vi "Calib_Analyse_fit.vi"(0 "Calib file":path, 1 "Input points":dbl[][](array[numeric]) format="%.2f", 2 "polynomial order":i32=2, 5 "Fixed n":bool=TRUE, 7 "n":dbl=0.45 format="%.2f", 9 "Point selector 3":cluster{"Y":dbl, "X":dbl, "t/f":bool}[](array[cluster]) {"X" format="%.2f"; "Y" format="%.2f"}, 11 "Point selector 4":T1(array[cluster])=[{"Y"=3.5155385742, "Y2"=3.2773117676, "X"=-15.0, "t/f"=FALSE}, {"Y"=3.4946367187, "Y2"=3.3075422363, "X"=-10.0, "t/f"=FALSE}, {"Y"=3.473232666, "Y2"=3.3353713379, "X"=-5.0, "t/f"=FALSE}, {"Y"=3.454592041, "Y2"=3.3658986816, "X"=0.0, "t/f"=FALSE}, {"Y"=3.4246572266, "Y2"=3.3874455566, "X"=5.0, "t/f"=FALSE}, {"Y"=3.398965332, "Y2"=3.4137351074, "X"=10.0, "t/f"=FALSE}, {"Y"=3.362712646484375, "Y2"=3.428485595703125, "X"=15.0, "t/f"=FALSE}] {"Y2" format="%.2f"; "X" format="%.2f"; "Y" format="%.2f"}) -> (4 "Calib const":string[][](array[string])=[["n", "0.405000"], ["A", "7.730378"], ["B", "6.204067"], ["Av % err", "0.204301"]], 6 "Calibration plot":cluster{cluster{dbl, dbl}[]}[](graph)=[{[{0.8450215822560672, 12.972948762710196}, {0.9063644870167936, 13.35352428024258}, {1.0129933166229186, 14.015056729178777}, {1.0924501688964157, 14.50801239851709}, {1.2215481063301497, 15.308944707524116}, {1.3521910897315237, 16.119462585897956}, {1.4772434835777744, 16.895296069694275}]}, {[{0.8450215822560672, 12.97084622363197}, {0.9063644870167936, 13.353228276297402}, {1.0129933166229186, 14.026771757587431}, {1.0924501688964157, 14.499243467101884}, {1.2215481063301497, 15.307992219000921}, {1.3521910897315237, 16.116882250583185}, {1.4772434835777744, 16.898281339562185}]}], 8 "Average Temp":dbl=19.0 format="%.2f", 10 "Point selector 3 out":cluster{"Y":dbl, "X":dbl, "t/f":bool}[](array[cluster]) {"X" format="%.2f"; "Y" format="%.2f"}, 14 "Coefficients":dbl[][](array[numeric]) format="%.2f", 15 "Point selector 4 out":T1(array[cluster])=[{"Y"=3.5155385742, "Y2"=3.2773117676, "X"=-15.0, "t/f"=FALSE}, {"Y"=3.4946367187, "Y2"=3.3075422363, "X"=-10.0, "t/f"=FALSE}, {"Y"=3.473232666, "Y2"=3.3353713379, "X"=-5.0, "t/f"=FALSE}, {"Y"=3.454592041, "Y2"=3.3658986816, "X"=0.0, "t/f"=FALSE}, {"Y"=3.4246572266, "Y2"=3.3874455566, "X"=5.0, "t/f"=FALSE}, {"Y"=3.398965332, "Y2"=3.4137351074, "X"=10.0, "t/f"=FALSE}, {"Y"=3.362712646484375, "Y2"=3.428485595703125, "X"=15.0, "t/f"=FALSE}] {"Y2" format="%.2f"; "X" format="%.2f"; "Y" format="%.2f"})   [LabVIEW 2010]
uses:
  Globals/Calib_global.vi
  Acquisition/PWA/PWAtasksGLOBAL.vi
  <vilib>/Analysis/NI_AALBase.lvlib
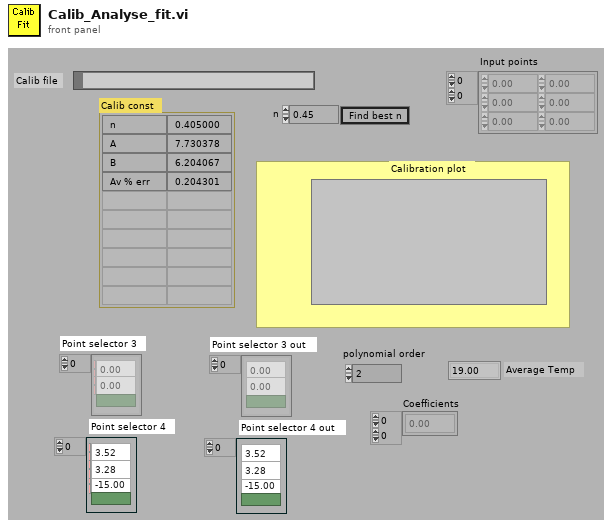
[diagram p1: front panel]
types:
  T1 = cluster{"Y":dbl, "Y2":dbl, "X":dbl, "t/f":bool}[]
  T2 = typedef "Cal_Inst_type.ctl" = enum16{"Propeller anemometer", "Pressure Transducer", "Hot wire", "Cross wire velocity", "Cross wire angle", "Generic Linear", "Generic Polynomial", "Generic BackPoly", "Fast FID", "Thermocouple", "Cold wire", "Pulsed Wire"}
  T3 = cluster{"Y":dbl, "Y":dbl, "X":dbl, "switch":bool}
  T4 = typedef "Ref_Inst_type.ctl" = enum16{"Propellor anemometer", "Pressure Transducer", "Raw voltage", "Pitot-static tube", "Preston tube", "Generic Linear", "Generic Polynomial", "Thermocouple", "LDA", "Enter Value", "ADAM Channel"}
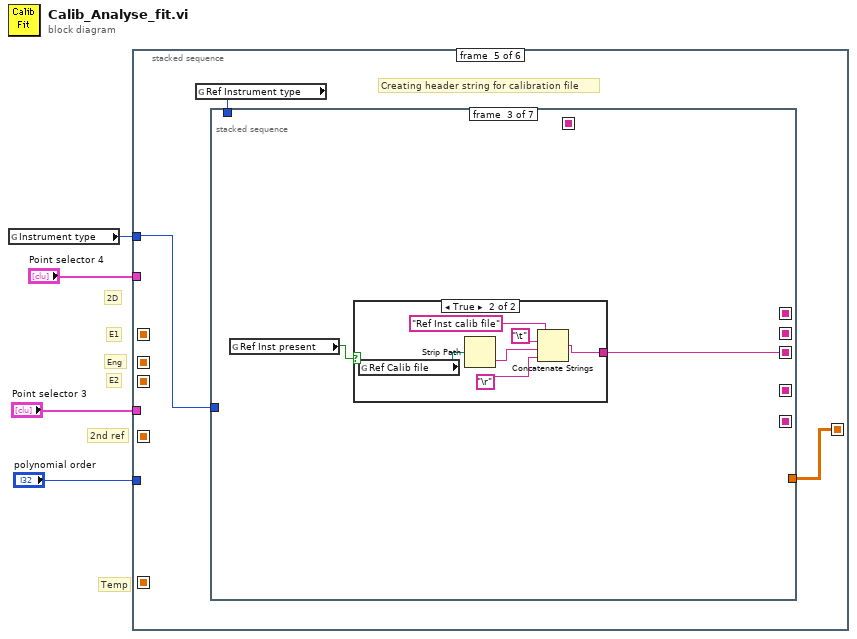
[diagram p0: block diagram]
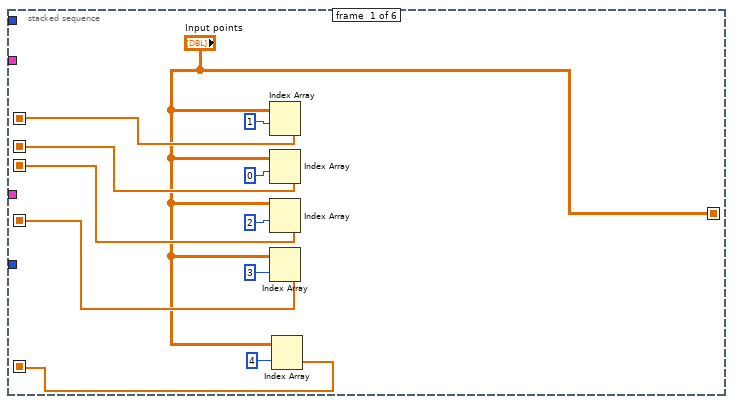
[diagram p2: hidden frame]
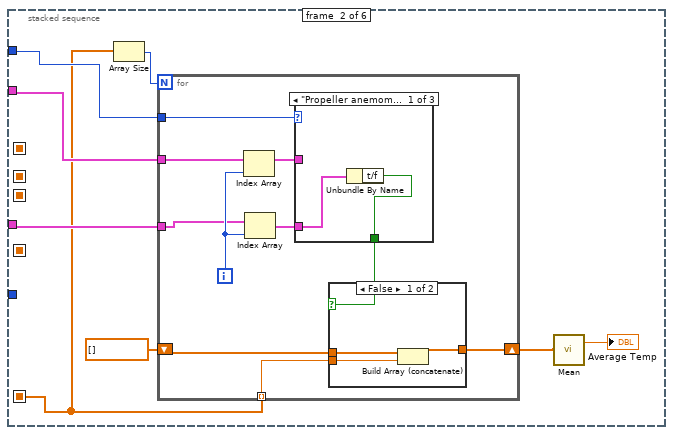
[diagram p3: hidden frame]
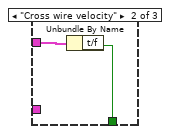
[diagram p5: hidden frame]
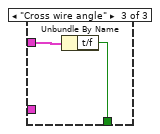
[diagram p6: hidden frame]
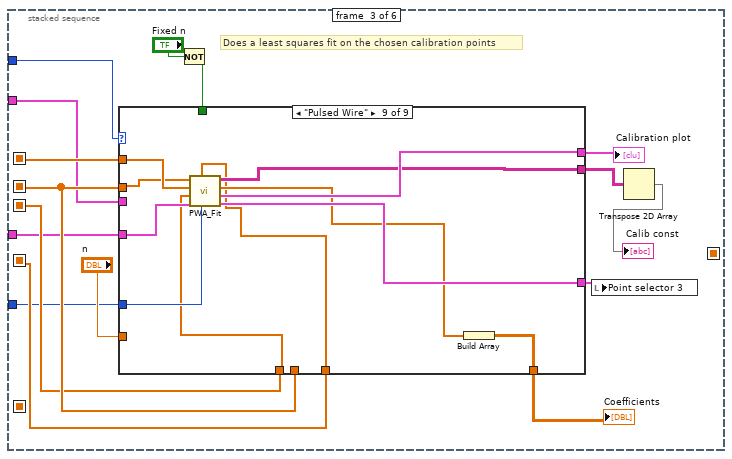
[diagram p7: hidden frame]
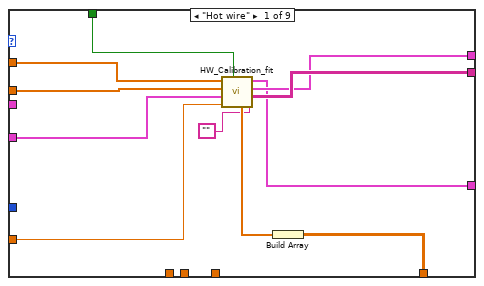
[diagram p8: hidden frame]
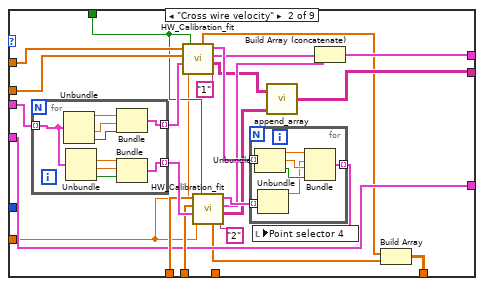
[diagram p9: hidden frame]
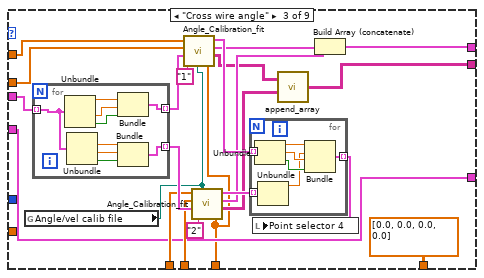
[diagram p10: hidden frame]
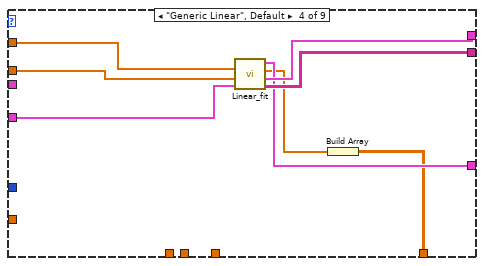
[diagram p11: hidden frame]
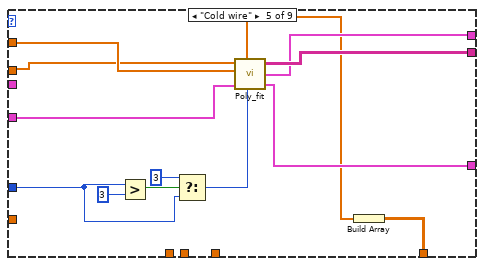
[diagram p12: hidden frame]
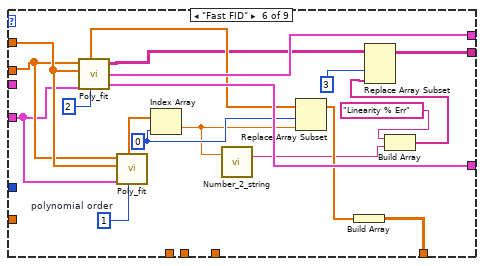
[diagram p13: hidden frame]
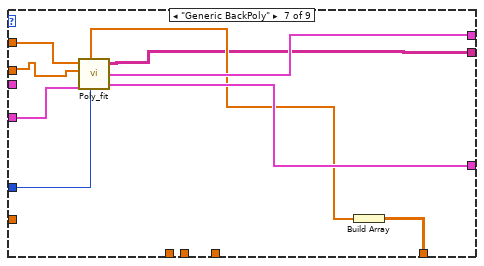
[diagram p14: hidden frame]
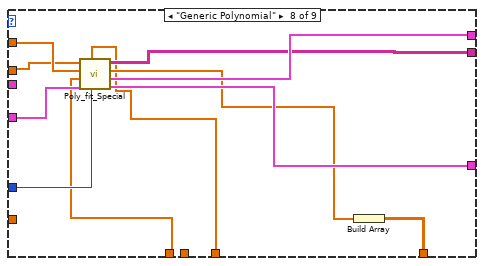
[diagram p15: hidden frame]
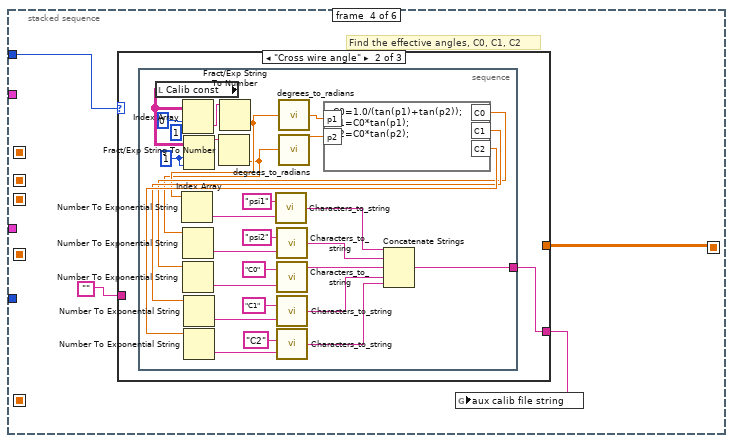
[diagram p16: hidden frame]
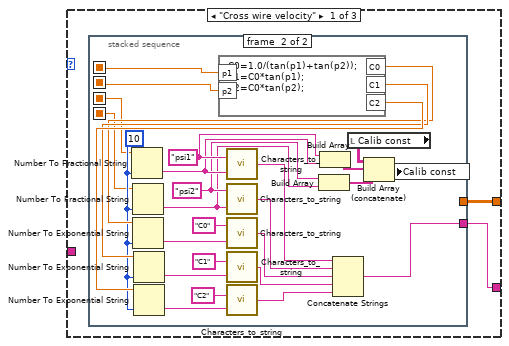
[diagram p17: hidden frame]
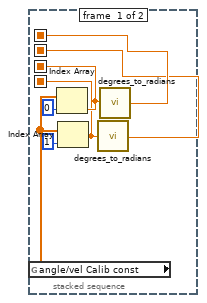
[diagram p18: hidden frame]
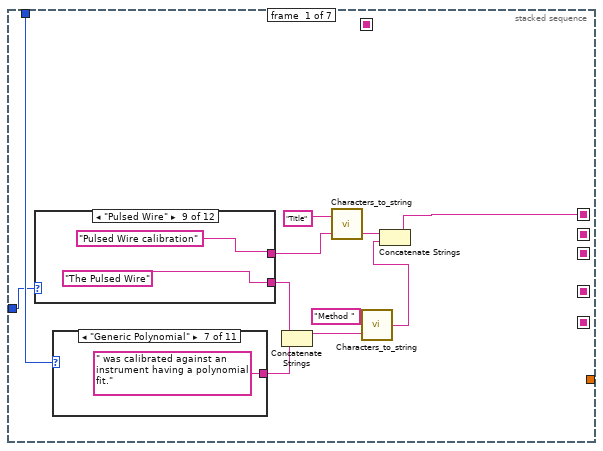
[diagram p20: hidden frame]
diagram:
  # "Temp"
  # "2D"
  # "2nd ref"
  # "E2"
  # "E1"
  # "Eng"
  n1 = global read "Calib_global.vi" "Instrument type"() -> (w4:T2)
  n2 = stacked-sequence {
    seq-local: ["Input points" _ _ _ _ _] -> [_ _ _ w221 w293 _]
    seq-local: [w11 _ _ _ _ _] -> [_ _ w52 _ _ _]
    seq-local: [w10 _ _ _ _ _] -> [_ _ w51 _ _ _]
    seq-local: [w9 _ _ _ _ _] -> [_ _ w50 _ _ _]
    seq-local: [w8 _ _ _ _ _] -> [_ _ w49 _ _ _]
    seq-local: [w5 _ _ _ _ _] -> [_ w17 _ _ _ _]
    tunnel: w4 -> [_ w23 w46 w220 w292 _]
    tunnel: "Point selector 3" -> [_ w22 w48 _ _ _]
    tunnel: "Point selector 4" -> [_ w21 w47 _ _ _]
    tunnel: "polynomial order" -> [_ _ w44 _ _ _]
    frame #0 {
      n3 = Index Array(array="Input points", index (row)=1) -> (element=w11:dbl[])  [unwired: 1 in]
      n4 = Index Array(array="Input points", index (row)=0) -> (element=w10:dbl[])  [unwired: 1 in]
      n5 = Index Array(array="Input points", index (row)=2) -> (element=w9:dbl[])  [unwired: 1 in]
      n6 = Index Array(array="Input points", index (row)=3) -> (element=w8:dbl[])  [unwired: 1 in]
      n7 = Index Array(array="Input points", index (row)=4) -> (element=w5:dbl[])  [unwired: 1 in]
    }
    frame #1 {
      n8 = Array Size(array=w17) -> (size(s)=w16:i32)
      n9 = for {
        N: w16 -> [_]
        tunnel: w23 -> [w33]
        tunnel: w22 -> [w25]
        tunnel: w21 -> [w27]
        shift-right: [w30] -> w18
        shift-left: dbl[] [] -> [w31]
        tunnel: w17 -> [w29] mode=indexing
        i -> [w26]
        n10 = Index Array(array=w27, index=w26) -> (element=w28:cluster{"Y":dbl, "Y2":dbl, "X":dbl, "t/f":bool})
        n11 = Index Array(array=w25, index=w26) -> (element=w24:cluster{"Y":dbl, "X":dbl, "t/f":bool})
        n12 = case shown="\"Propeller anemometer\", Default" w33 {
          tunnel: w24 -> [w39 _ _]
          tunnel: w28 -> [_ w41 w43]
          tunnel: [w38 w40 w42] -> w32
          frame "Propeller anemometer", Default {
            n13 = Unbundle By Name(w39) -> ("t/f"=w38:bool)
          }
          frame "Cross wire velocity" {
            n14 = Unbundle By Name(w41) -> ("t/f"=w40:bool)
          }
          frame "Cross wire angle" {
            n15 = Unbundle By Name(w43) -> ("t/f"=w42:bool)
          }
        }
        n16 = case shown="False" w32 {
          tunnel: w31 -> [w36 w37]
          tunnel: [w35 w37] -> w30
          tunnel: w29 -> [w34 _]
          frame False {
            n17 = Build Array (concatenate)(w36, w34) -> (w35:dbl[])
          }
          frame True {
          }
        }
      }
      n18 = call <vilib>:"Mean.vi"("X"=w18) -> ("mean"=→"Average Temp":dbl)  [unwired: 1 out]
    }
    frame #2 {
      # "Does a least squares fit on the chosen calibration points"
      n19 = Not(x="Fixed n") -> (.not. x?=w54:bool)
      n20 = case shown="\"Pulsed Wire\"" w46 {
        tunnel: [w65 w82 w120 w151 w166 w187 w196 w207 w218] -> w57
        tunnel: w52 -> [w70 w94 w132 w156 w165 w176 w193 w205 w216]
        tunnel: w51 -> [w69 w93 w131 w155 w164 w175 w192 w204 w215]
        tunnel: w54 -> [w68 w80 _ _ _ _ _ _ _]
        tunnel: w47 -> [_ w83 w121 _ _ _ _ _ _]
        tunnel: [w67 w76 w114 w154 w169 w177 w190 w201 w212] -> w55
        tunnel: [w66 w84 w122 w153 w168 w188 w197 w208 w219] -> w56
        tunnel: w51 -> [_ w89 w127 _ _ _ _ _ _]
        tunnel: w50 -> [_ w88 w126 _ _ _ _ w199 w210]
        tunnel: w48 -> [w64 w82 w120 w152 w167 w174 w194 w203 w214]
        tunnel: "n" -> [w63 w79 _ _ _ _ _ _ _]
        tunnel: w49 -> [_ _ w113 _ _ _ _ w198 w209]
        tunnel: [w61 w73 dbl[][] [[0.0, 0.0], [0.0, 0.0]] w149 w158 w186 w195 w206 w217] -> w45
        tunnel: w44 -> [_ _ _ _ w157 _ w189 w200 w211]
        frame "Hot wire" {
          n21 = call "HW_Calibration_fit.vi"("coeff suffix"="", "Fixed n (F)"=w68, "n input  (0.45)"=w63, "Point selector"=w64, "Velocity"=w69, "HW voltage"=w70) -> ("Calib const"=w67:string[][], "Calibration plot"=w66:cluster{cluster{dbl, "mse":dbl}[]}[], "Point selector"=w65:cluster{"Y":dbl, "X":dbl, "switch":bool}[], "Coefficients"=w62:dbl[])
          n22 = Build Array(w62) -> (w61:dbl[][])
        }
        frame "Cross wire velocity" {
          n23 = for {
            tunnel: w83 -> [w106] mode=indexing
            tunnel: [w107] -> w92 mode=indexing
            tunnel: [w105] -> w90 mode=indexing
            n24 = Unbundle(w106) -> ("Y"=w110:dbl, "X"=w109:dbl, "t/f"=w108:bool)  [unwired: 1 out]
            n25 = Unbundle(w106) -> ("Y2"=w104:dbl, "X"=w103:dbl, "t/f"=w102:bool)  [unwired: 1 out]
            n26 = Bundle("Y"=w110, "X"=w109, "t/f"=w108) -> (w107:cluster{"Y":dbl, "X":dbl, "t/f":bool})  [unwired: 1 out]
            n27 = Bundle("Y2"=w104, "X"=w103, "t/f"=w102) -> (w105:cluster{"Y2":dbl, "X":dbl, "t/f":bool})  [unwired: 1 out]
          }
          n28 = call "HW_Calibration_fit.vi"("coeff suffix"="1", "Fixed n (F)"=w80, "n input  (0.45)"=w79, "Point selector"=w92, "Velocity"=w93, "HW voltage"=w94) -> ("Calib const"=w77:string[][], "Calibration plot"=w85:cluster{cluster{dbl, "mse":dbl}[]}[], "Point selector"=w91:cluster{"Y":dbl, "X":dbl, "switch":bool}[], "Coefficients"=w71:dbl[])
          n29 = call "HW_Calibration_fit.vi"("coeff suffix"="2", "Fixed n (F)"=w80, "n input  (0.45)"=w79, "Point selector"=w90, "Velocity"=w89, "HW voltage"=w88) -> ("Calib const"=w78:string[][], "Calibration plot"=w86:cluster{cluster{dbl, "mse":dbl}[]}[], "Point selector"=w87:cluster{"Y":dbl, "X":dbl, "switch":bool}[], "Coefficients"=w72:dbl[])
          n30 = for {
            tunnel: w91 -> [w101] mode=indexing
            tunnel: [w97] -> w81 mode=indexing
            tunnel: w87 -> [w96] mode=indexing
            n31 = Unbundle(w101) -> ("Y"=w100:dbl, "X"=w99:dbl, "switch"=w98:bool)
            n32 = Unbundle(w96) -> ("Y"=w95:dbl)  [unwired: 2 out]
            n33 = Bundle("Y"=w100, "Y"=w95, "X"=w99, "switch"=w98) -> (w97:T3)  [unwired: 1 out]
          }
          n34 = local write "Point selector 4"(w81) -> ()
          n35 = call "append_array.vi"("array 2"=w78, "array 1"=w77) -> ("appended array"=w76:string[][])
          n36 = Build Array (concatenate)(w85, w86) -> (w84:cluster{cluster{dbl, "mse":dbl}[]}[])
          n37 = Build Array(w71, w72) -> (w73:dbl[][])
        }
        frame "Cross wire angle" {
          n38 = global read "Calib_global.vi" "Angle/vel calib file"() -> (w112:path)
          n39 = for {
            tunnel: w121 -> [w144] mode=indexing
            tunnel: [w145] -> w130 mode=indexing
            tunnel: [w143] -> w128 mode=indexing
            n40 = Unbundle(w144) -> ("Y"=w148:dbl, "X"=w147:dbl, "t/f"=w146:bool)  [unwired: 1 out]
            n41 = Unbundle(w144) -> ("Y2"=w142:dbl, "X"=w141:dbl, "t/f"=w140:bool)  [unwired: 1 out]
            n42 = Bundle("Y"=w148, "X"=w147, "t/f"=w146) -> (w145:cluster{"Y":dbl, "X":dbl, "t/f":bool})  [unwired: 1 out]
            n43 = Bundle("Y2"=w142, "X"=w141, "t/f"=w140) -> (w143:cluster{"Y2":dbl, "X":dbl, "t/f":bool})  [unwired: 1 out]
          }
          n44 = call "Angle_Calibration_fit.vi"("Reference Velocity"=w113, "Vel calib file"=w112, "coeff suffix"="1", "Point selector"=w130, "Angle"=w131, "HW voltage"=w132) -> ("Calib const"=w116:string[][], "Angle calibration (output)"=w123:cluster{cluster{"Y":dbl, "Y":dbl}[]}[], "Point selector"=w129:cluster{"Y":dbl, "X":dbl, "switch":bool}[])
          n45 = call "Angle_Calibration_fit.vi"("Reference Velocity"=w113, "Vel calib file"=w112, "coeff suffix"="2", "Point selector"=w128, "Angle"=w127, "HW voltage"=w126) -> ("Calib const"=w115:string[][], "Angle calibration (output)"=w124:cluster{cluster{"Y":dbl, "Y":dbl}[]}[], "Point selector"=w125:cluster{"Y":dbl, "X":dbl, "switch":bool}[])
          n46 = for {
            tunnel: w129 -> [w139] mode=indexing
            tunnel: [w135] -> w119 mode=indexing
            tunnel: w125 -> [w134] mode=indexing
            n47 = Unbundle(w139) -> ("Y"=w138:dbl, "X"=w137:dbl, "switch"=w136:bool)
            n48 = Unbundle(w134) -> ("Y"=w133:dbl)  [unwired: 2 out]
            n49 = Bundle("Y"=w138, "Y"=w133, "X"=w137, "switch"=w136) -> (w135:T3)  [unwired: 1 out]
          }
          n50 = local write "Point selector 4"(w119) -> ()
          n51 = call "append_array.vi"("array 2"=w115, "array 1"=w116) -> ("appended array"=w114:string[][])
          n52 = Build Array (concatenate)(w123, w124) -> (w122:cluster{cluster{"Y":dbl, "Y":dbl}[]}[])
        }
        frame "Generic Linear", Default {
          n53 = call "Linear_fit.vi"("Point selector"=w152, "Input X array"=w155, "Input Y array"=w156) -> ("Calib const"=w154:string[][], "Calibration plot"=w153:cluster{cluster{dbl, dbl}[]}[], "Coefficients"=w150:dbl[], "Point selector"=w151:cluster{"Y":dbl, "X":dbl, "switch":bool}[])  [unwired: 1 out]
          n54 = Build Array(w150) -> (w149:dbl[][])
        }
        frame "Cold wire" {
          n55 = Greater?(x=w157, y=3) -> (0:w162:bool)
          n56 = Select(t=3, s=w162, f=w157) -> (s? t:f=w160:i32)
          n57 = call "Poly_fit.vi"("Input Y array"=w164, "Input X array"=w165, "polynomial order"=w160, "Point selector"=w167) -> ("Coefficients"=w159:dbl[], "Calib const"=w169:string[][], "Calibration plot"=w168:cluster{cluster{dbl, dbl}[]}[], "Point selector"=w166:cluster{"Y":dbl, "X":dbl, "switch":bool}[])  [unwired: 1 out]
          n58 = Build Array(w159) -> (w158:dbl[][])
        }
        frame "Fast FID" {
          w181 = 0 ("index")
          w184 = 1  # polynomial order
          n59 = call "Poly_fit.vi"("Input Y array"=w175, "Input X array"=w176, "polynomial order"=2, "Point selector"=w174) -> ("Coefficients"=w182:dbl[], "Calib const"=w179:string[][], "Calibration plot"=w188:cluster{cluster{dbl, dbl}[]}[], "Point selector"=w187:cluster{"Y":dbl, "X":dbl, "switch":bool}[])  [unwired: 1 out]
          n60 = call "Poly_fit.vi"("Input Y array"=w175, "Input X array"=w176, "polynomial order"=w184, "Point selector"=w174) -> ("Coefficients"=w183:dbl[])  [unwired: 4 out]
          n61 = Index Array(array=w183, index=w181) -> (element=w173:dbl)
          n62 = call "Number_2_string.vi"("number"=w173) -> ("String"=w171:string)  [unwired: 1 in]
          n63 = Replace Array Subset(array=w182, new element=w173, index=w181) -> (w180:dbl[])
          n64 = Build Array(w180) -> (w186:dbl[][])
          n65 = Build Array("Linearity % Err" ("new element/subarray"), w171) -> (w170:string[])
          n66 = Replace Array Subset(array=w179, new element=w170, index (col)=3 ("disabled index (col)")) -> (w177:string[][])  [unwired: 1 in]
        }
        frame "Generic BackPoly" {
          n67 = call "Poly_fit.vi"("Input Y array"=w193, "Input X array"=w192, "polynomial order"=w189, "Point selector"=w194) -> ("Coefficients"=w191:dbl[], "Calib const"=w190:string[][], "Calibration plot"=w197:cluster{cluster{dbl, dbl}[]}[], "Point selector"=w196:cluster{"Y":dbl, "X":dbl, "switch":bool}[])  [unwired: 1 out]
          n68 = Build Array(w191) -> (w195:dbl[][])
        }
        frame "Generic Polynomial" {
          n69 = call "Poly_fit_Special.vi"("polynomial order"=w200, "Input X^3"=w198, "Point selector"=w203, "Input X^2"=w199, "Input X array"=w205, "Input Y array"=w204) -> ("Point selector"=w207:cluster{"Y":dbl, "X":dbl, "switch":bool}[], "Calibration plot"=w208:cluster{cluster{dbl, dbl}[]}[], "Coefficients"=w202:dbl[], "Calib const"=w201:string[][])
          n70 = Build Array(w202) -> (w206:dbl[][])
        }
        frame "Pulsed Wire" {
          n71 = call "PWA_Fit.vi"("polynomial order"=w211, "Input X^3"=w209, "Point selector"=w214, "Input X^2"=w210, "Input X array"=w216, "Input Y array"=w215) -> ("Point selector"=w218:cluster{"Y":dbl, "X":dbl, "switch":bool}[], "Calibration plot"=w219:cluster{cluster{dbl, dbl}[]}[], "Coefficients"=w213:dbl[], "Calib const"=w212:string[][])
          n72 = Build Array(w213) -> (w217:dbl[][])
        }
      }
      "Calibration plot" <- w56
      "Coefficients" <- w45
      n73 = local write "Point selector 3"(w57) -> ()
      n74 = Transpose 2D Array(2D array=w55) -> (transposed array=→"Calib const":string[][])
    }
    frame #3 {
      # "Find the effective angles, C0, C1, C2"
      n75 = case shown="\"Cross wire angle\"" w220 {
        tunnel: "" -> [_ _ w291]
        tunnel: [w225 w261 w291] -> w223
        tunnel: w221 -> [w224 _ _]
        frame "Cross wire velocity" {
          n76 = stacked-sequence {
            seq-local: [w230 _] -> [_ w236]
            seq-local: [w229 _] -> [_ w234]
            seq-local: [w228 _] -> [_ w235]
            seq-local: [w227 _] -> [_ w233]
            tunnel: [_ w246] -> w225
            tunnel: w224 -> [_ _]
            frame #0 {
              n77 = global read "Calib_global.vi" "angle/vel Calib const"() -> (w226:dbl[])
              n78 = Index Array(array=w226, index=0) -> (element=w228:dbl)
              n79 = Index Array(array=w226, index=1) -> (element=w227:dbl)
              n80 = call "degrees_to_radians.vi"("degrees"=w227) -> ("radians"=w229:dbl)
              n81 = call "degrees_to_radians.vi"("degrees"=w228) -> ("radians"=w230:dbl)
            }
            frame #1 {
              w237 = 10
              w243 = "psi2"
              w245 = "psi1"
              n82 = Number To Fractional String(number=w235, precision (6)=w237) -> (F-format string=w244:string)  [unwired: 2 out]
              n83 = Number To Fractional String(number=w233, precision (6)=w237) -> (F-format string=w242:string)  [unwired: 2 out]
              n84 = formula code="C0=1.0/(tan(p1)+tan(p2));\nC1=C0*tan(p1);\nC2=C0*tan(p2);"("p1"=w236, "p2"=w234) -> ("C0"=w258:dbl, "C1"=w259:dbl, "C2"=w260:dbl)
              n85 = Number To Exponential String(number=w258, precision (6)=w237) -> (E-format string=w256:string)  [unwired: 2 out]
              n86 = Number To Exponential String(number=w259, precision (6)=w237) -> (E-format string=w254:string)  [unwired: 2 out]
              n87 = Number To Exponential String(number=w260, precision (6)=w237) -> (E-format string=w252:string)  [unwired: 2 out]
              n88 = call "Characters_to_string.vi"("Characters to write"=w244, "Label for characters"=w245) -> ("Output string"=w250:string)
              n89 = call "Characters_to_string.vi"("Characters to write"=w242, "Label for characters"=w243) -> ("Output string"=w249:string)
              n90 = call "Characters_to_string.vi"("Characters to write"=w256, "Label for characters"="C0") -> ("Output string"=w251:string)
              n91 = call "Characters_to_string.vi"("Characters to write"=w254, "Label for characters"="C1") -> ("Output string"=w248:string)
              n92 = call "Characters_to_string.vi"("Characters to write"=w252, "Label for characters"="C2") -> ("Output string"=w247:string)
              n93 = Build Array(w243, w242) -> (w240:string[])
              n94 = Build Array(w245, w244) -> (w241:string[])
              n95 = Concatenate Strings(w250, w249, w251, w248, w247) -> (w246:string)
              n96 = local read "Calib const"() -> (w239:string[][])
              n97 = Build Array (concatenate)(w239, w241, w240) -> (w238:string[][])
              n98 = local write "Calib const"(w238) -> ()
            }
          }
        }
        frame "Cross wire angle" {
          n99 = stacked-sequence {
            tunnel: [w272] -> w261
            frame #0 {
              w271 = 1
              n100 = local read "Calib const"() -> (w269:string[][])
              n101 = Index Array(array=w269, index (row)=0, index (col)=1) -> (element=w268:string)
              n102 = Index Array(array=w269, index (row)=w271, index (col)=w271) -> (element=w267:string)
              n103 = Fract/Exp String To Number(string=w267) -> (number=w262:dbl)  [unwired: 4 out]
              n104 = Number To Exponential String(number=w262) -> (E-format string=w284:string)  [unwired: 3 out]
              n105 = Fract/Exp String To Number(string=w268) -> (number=w265:dbl)  [unwired: 4 out]
              n106 = Number To Exponential String(number=w265) -> (E-format string=w285:string)  [unwired: 3 out]
              n107 = call "Characters_to_string.vi"("Characters to write"=w285, "Label for characters"="psi1") -> ("Output string"=w276:string)
              n108 = call "Characters_to_string.vi"("Characters to write"=w284, "Label for characters"="psi2") -> ("Output string"=w275:string)
              n109 = call "degrees_to_radians.vi"("degrees"=w265) -> ("radians"=w264:dbl)
              n110 = call "degrees_to_radians.vi"("degrees"=w262) -> ("radians"=w263:dbl)
              n111 = formula code="C0=1.0/(tan(p1)+tan(p2));\nC1=C0*tan(p1);\nC2=C0*tan(p2);"("p1"=w264, "p2"=w263) -> ("C0"=w288:dbl, "C1"=w289:dbl, "C2"=w290:dbl)
              n112 = Number To Exponential String(number=w288) -> (E-format string=w282:string)  [unwired: 3 out]
              n113 = Number To Exponential String(number=w289) -> (E-format string=w280:string)  [unwired: 3 out]
              n114 = Number To Exponential String(number=w290) -> (E-format string=w278:string)  [unwired: 3 out]
              n115 = call "Characters_to_string.vi"("Characters to write"=w282, "Label for characters"="C0") -> ("Output string"=w277:string)
              n116 = call "Characters_to_string.vi"("Characters to write"=w280, "Label for characters"="C1") -> ("Output string"=w274:string)
              n117 = call "Characters_to_string.vi"("Characters to write"=w278, "Label for characters"="C2") -> ("Output string"=w273:string)
              n118 = Concatenate Strings(w276, w275, w277, w274, w273) -> (w272:string)
            }
          }
        }
        frame "Generic Linear", Default {
        }
      }
      n119 = global write "Calib_global.vi" "aux calib file string"(w223) -> ()
    }
    frame #4 {
      # "Creating header string for calibration file"
      n120 = global read "Calib_global.vi" "Ref Instrument type"() -> (w294:T4)
      n121 = stacked-sequence {
        seq-local: [_ w355 _ _ _ _ _] -> [_ _ _ _ _ _ w650]
        seq-local: [w303 _ _ _ _ _ _] -> [_ _ _ _ _ _ w651]
        seq-local: [_ _ w364 _ _ _ _] -> [_ _ _ _ _ _ w649]
        seq-local: [_ _ _ w378 _ _ _] -> [_ _ _ _ _ _ w646]
        seq-local: [_ _ _ _ _ w629 _] -> [_ _ _ _ _ _ w647]
        seq-local: [_ _ _ _ w483 _ _] -> [_ _ _ _ _ w630 _]
        tunnel: w294 -> [w298 _ _ _ _ _ _]
        tunnel: w293 -> [_ _ _ _ w480 _ _]
        tunnel: w292 -> [w295 w348 _ w376 w474 w628 w652]
        frame #0 {
          n122 = case shown="\"Pulsed Wire\"" w295 {
            tunnel: ["Propeller Anemometer velocity calibration" "Pressure Transducer calibration" "Hot wire velocity calibration" "Cross wire velocity calibration" "Cross wire angle calibration" "Fast FID calibration" "Generic Linear calibration" "Generic Polynomial calibration" "Pulsed Wire calibration" "Generic Backwards Polynomial calibration" "Thermocouple calibration" "Cold wire calibration"] -> w302
            tunnel: ["The Propeller Anemometer" "The Pressure Transducer" "The Hot wire" "The Cross wire" "The Cross wire" "The Fast FID" "The Generic Linear Instrument" "The Generic Polynomial Instrument" "The Pulsed Wire" "The Generic Backwards Polynomial Instrument" "The Thermocouple" "The Cold wire"] -> w299
            frame "Propeller anemometer" {
            }
            frame "Pressure Transducer" {
            }
            frame "Hot wire" {
            }
            frame "Cross wire velocity" {
            }
            frame "Cross wire angle" {
            }
            frame "Fast FID" {
            }
            frame "Generic Linear" {
            }
            frame "Generic Polynomial" {
            }
            frame "Pulsed Wire" {
            }
            frame "Generic BackPoly" {
            }
            frame "Thermocouple" {
            }
            frame "Cold wire" {
            }
          }
          n123 = case shown="\"Generic Polynomial\"" w298 {
            tunnel: [" was calibrated for velocity against a Propeller Anemometer." " was calibrated for pressure against a Pressure Transducer." " was calibrated against a voltage" " was calibrated for velocity against a Pitot-static tube." " was calibrated against a Preston tube." " was calibrated against an instrument having a Linear fit." " was calibrated against an instrument having a polynomial fit." " was calibrated for temperature against a thermocouple." " was calibrated for velocity against the LDA." " was calibrated against the reading entered by the user." " was calibrated against an ADAM channel."] -> w300
            frame "Propellor anemometer" {
            }
            frame "Pressure Transducer" {
            }
            frame "Raw voltage" {
            }
            frame "Pitot-static tube" {
            }
            frame "Preston tube" {
            }
            frame "Generic Linear" {
            }
            frame "Generic Polynomial" {
            }
            frame "Thermocouple" {
            }
            frame "LDA" {
            }
            frame "Enter Value" {
            }
            frame "ADAM Channel" {
            }
          }
          n124 = Concatenate Strings(w299, w300) -> (w297:string)
          n125 = call "Characters_to_string.vi"("Characters to write"=w302, "Label for characters"="Title") -> ("Output string"=w304:string)
          n126 = call "Characters_to_string.vi"("Characters to write"=w297, "Label for characters"="Method ") -> ("Output string"=w296:string)
          n127 = Concatenate Strings(w304, w296) -> (w303:string)
        }
        frame #1 {
          n128 = local read "Average Temp"() -> (w347:dbl)
          n129 = case shown="\"Cross wire angle\"" w348 {
            tunnel: [w360 ""] -> w351
            frame "Cross wire angle" {
              n130 = global read "Calib_global.vi" "Angle/vel calib file"() -> (w359:path)
              n131 = Strip Path(path=w359) -> (name=w358:string)  [unwired: 1 out]
              n132 = call "Characters_to_string.vi"("Characters to write"=w358, "Label for characters"="Original vel calib") -> ("Output string"=w360:string)
            }
            frame "Generic Linear", Default {
            }
          }
          n133 = global read "Calib_global.vi" "Abs Press (mbar)"() -> (w350:dbl)
          n134 = Strip Path(path="Calib file") -> (name=w345:string)  [unwired: 1 out]
          n135 = call "Characters_to_string.vi"("Characters to write"="Calibration_File", "Label for characters"="File_Type") -> ("Output string"=w341:string)
          n136 = call "Value_to_string.vi"("Value"=w347, "Label for value"="Calib temp") -> ("Output string"=w352:string)  [unwired: 1 in]
          n137 = call "Value_to_string.vi"("Value"=w350, "Label for value"="Abs Press (mbar)") -> ("Output string"=w353:string)  [unwired: 1 in]
          n138 = call "Characters_to_string.vi"("Characters to write"=w345, "Label for characters"="File name") -> ("Output string"=w342:string)
          n139 = call "Date_and_Time_to_string.vi"() -> ("Date and time (spreadsheet)"=w354:string)
          n140 = Concatenate Strings(w354, w342, w341, w351, w352, w353) -> (w355:string)
        }
        frame #2 {
          n141 = global read "Calib_global.vi" "Ref Inst present"() -> (w363:bool)
          n142 = case shown="True" w363 {
            tunnel: ["" w371] -> w364
            frame False {
            }
            frame True {
              n143 = global read "Calib_global.vi" "Ref Calib file"() -> (w367:path)
              n144 = Strip Path(path=w367) -> (name=w366:string)  [unwired: 1 out]
              n145 = Concatenate Strings("Ref Inst calib file", "\t", w366, "\r") -> (w371:string)
            }
          }
        }
        frame #3 {
          n146 = local read "Calib const"() -> (w372:string[][])
          n147 = Index Array(array=w372, index (col)=1) -> (element=w374:string[])  [unwired: 1 in]
          n148 = case shown="\"Pulsed Wire\"" w376 {
            tunnel: [w393 w406 w411 w420 w433 w444 w456 w462 w473] -> w377
            tunnel: w374 -> [_ _ w414 w423 w436 w447 _ _ _]
            tunnel: [2 ("Index") 3 ("Index") 6 ("Index") 9 ("Index") 6 ("Index") 4 ("Index") 3 ("Index") 2 ("Index") 7 ("Index")] -> w375
            tunnel: ["Av % Err" "Linearity % Err" "Av % Err" "Av % err -ve" "Av % Err" "Av % Err" "Av % Err" "Av % Err" "Av % Err"] -> w373
            tunnel: w372 -> [_ _ _ w425 _ _ _ _ _]
            frame "Propeller anemometer", Default {
              n149 = Build Array("Coeff A", "Coeff B") -> (w393:string[])
            }
            frame "Fast FID" {
              n150 = Build Array("Coeff A", "Coeff B", "Coeff C", "Fast FID Bkgnd", "Fast FID Bkgnd Variance", "FFID Bkgnd Volts", "FFID Bkgnd Time", "FFID Bkgnd Filename") -> (w406:string[])
            }
            frame "Generic Polynomial" {
              n151 = Array Size(array=w414) -> (size(s)=w415:i32)
              n152 = Decrement(x=w415) -> (x-1=w413:i32)
              n153 = Build Array("Coeff A", "Coeff B", "Coeff C", "Coeff D", "Coeff E", "Coeff F") -> (w412:string[])
              n154 = Array Subset(array=w412, length=w413) -> (w411:string[])  [unwired: 1 in]
            }
            frame "Pulsed Wire" {
              n155 = Array Size(array=w423) -> (size(s)=w424:i32)
              n156 = Index Array(array=w425, index (col)=0) -> (element=w422:string[])  [unwired: 1 in]
              n157 = Decrement(x=w424) -> (x-1=w421:i32)
              n158 = Array Subset(array=w422, length=w421) -> (w420:string[])  [unwired: 1 in]
            }
            frame "Generic BackPoly" {
              n159 = Array Size(array=w436) -> (size(s)=w437:i32)
              n160 = Decrement(x=w437) -> (x-1=w435:i32)
              n161 = Build Array("Coeff A", "Coeff B", "Coeff C", "Coeff D", "Coeff E", "Coeff F") -> (w434:string[])
              n162 = Array Subset(array=w434, length=w435) -> (w433:string[])  [unwired: 1 in]
            }
            frame "Cold wire" {
              n163 = Array Size(array=w447) -> (size(s)=w448:i32)
              n164 = Decrement(x=w448) -> (x-1=w446:i32)
              n165 = Build Array("Coeff A", "Coeff B", "Coeff C", "Coeff D") -> (w445:string[])
              n166 = Array Subset(array=w445, length=w446) -> (w444:string[])  [unwired: 1 in]
            }
            frame "Hot wire" {
              n167 = Build Array("Coeff n", "Coeff A", "Coeff B") -> (w456:string[])
            }
            frame "Cross wire angle" {
              n168 = Build Array("psi1", "psi2") -> (w462:string[])
            }
            frame "Cross wire velocity" {
              n169 = Build Array("Coeff n1", "Coeff A1", "Coeff B1", "Av % Err", "Coeff n2", "Coeff A2", "Coeff B2") -> (w473:string[])
            }
          }
          n170 = for {
            shift-right: [w389] -> w381
            shift-left: "\r" -> [w390]
            tunnel: w377 -> [w388] mode=indexing
            tunnel: w374 -> [w386]
            i -> [w387]
            n171 = Index Array(array=w386, index=w387) -> (element=w385:string)
            n172 = call "Characters_to_string.vi"("Characters to write"=w385, "Label for characters"=w388) -> ("Output string"=w384:string)
            n173 = Concatenate Strings(w390, w384) -> (w389:string)
          }
          n174 = Index Array(array=w374, index=w375) -> (element=w380:string)
          n175 = call "Characters_to_string.vi"("Characters to write"=w380, "Label for characters"=w373) -> ("Output string"=w382:string)
          n176 = Concatenate Strings(w381, w382) -> (w378:string)
        }
        frame #4 {
          n177 = local read "Point selector 3"() -> (w482:cluster{"Y":dbl, "X":dbl, "t/f":bool}[])
          n178 = local read "Point selector 4"() -> (w481:T1)
          n179 = case shown="\"Generic Polynomial\"" w474 {
            tunnel: [w488 w499 w510 w524 w537 w547 w562 w576 w586 w599 w609 w620] -> w484
            tunnel: w482 -> [w487 w498 w509 _ _ w546 w561 w575 w585 w598 w608 w619]
            tunnel: w481 -> [_ _ _ w522 w536 _ _ _ _ _ _ _]
            tunnel: [w486 w497 w508 w521 w533 w545 w560 w573 w584 w597 w607 w618] -> w478
            frame "Propeller anemometer" {
              n180 = for {
                tunnel: w487 -> [w496] mode=indexing
                tunnel: [w494] -> w486 mode=indexing
                n181 = Unbundle By Name(w496) -> ("t/f"=w495:bool)
                n182 = Select(t="NaN not included", s=w495, f="") -> (s? t:f=w494:string)
              }
              n183 = Concatenate Strings("Velocity m/s", "\t", "Voltage") -> (w488:string)
            }
            frame "Pressure Transducer" {
              n184 = for {
                tunnel: w498 -> [w505] mode=indexing
                tunnel: [w506] -> w497 mode=indexing
                n185 = Unbundle By Name(w505) -> ("t/f"=w507:bool)
                n186 = Select(t="NaN not included", s=w507, f="") -> (s? t:f=w506:string)
              }
              n187 = Concatenate Strings("Pressure mmH2O", "\t", "Voltage") -> (w499:string)
            }
            frame "Hot wire" {
              n188 = for {
                tunnel: w509 -> [w518] mode=indexing
                tunnel: [w516] -> w508 mode=indexing
                n189 = Unbundle By Name(w518) -> ("t/f"=w517:bool)
                n190 = Select(t="NaN not included", s=w517, f="") -> (s? t:f=w516:string)
              }
              n191 = Concatenate Strings("Velocity m/s", "\t", "Voltage") -> (w510:string)
            }
            frame "Cross wire velocity" {
              w523 = "\t"
              n192 = for {
                tunnel: w522 -> [w530] mode=indexing
                tunnel: [w529] -> w521 mode=indexing
                n193 = Unbundle By Name(w530) -> ("t/f"=w527:bool)
                n194 = Select(t="NaN not included", s=w527, f="") -> (s? t:f=w529:string)
              }
              n195 = Concatenate Strings("Velocity m/s", w523, "Voltage1", w523, "Voltage2") -> (w524:string)
            }
            frame "Cross wire angle" {
              w531 = "\t"
              n196 = for {
                tunnel: w536 -> [w543] mode=indexing
                tunnel: [w541] -> w533 mode=indexing
                n197 = Unbundle By Name(w543) -> ("t/f"=w542:bool)
                n198 = Select(t="NaN not included", s=w542, f="") -> (s? t:f=w541:string)
              }
              n199 = Concatenate Strings("Angle (degrees)", w531, "Voltage1", w531, "Voltage2", w531, "Ref velocity") -> (w537:string)
            }
            frame "Generic Linear" {
              n200 = global read "Calib_global.vi" "calib units"() -> (w544:string)
              n201 = for {
                tunnel: w546 -> [w554] mode=indexing
                tunnel: [w552] -> w545 mode=indexing
                n202 = Unbundle By Name(w554) -> ("t/f"=w553:bool)
                n203 = Select(t="NaN not included", s=w553, f="") -> (s? t:f=w552:string)
              }
              n204 = Concatenate Strings(w544, "\t", "Voltage") -> (w547:string)
            }
            frame "Generic Polynomial" {
              w558 = "\t"
              n205 = global read "Calib_global.vi" "calib units"() -> (w559:string)
              n206 = for {
                tunnel: w561 -> [w568] mode=indexing
                tunnel: [w566] -> w560 mode=indexing
                n207 = Unbundle By Name(w568) -> ("t/f"=w567:bool)
                n208 = Select(t="NaN not included", s=w567, f="") -> (s? t:f=w566:string)
              }
              n209 = Concatenate Strings(w559, w558, "Volts", w558, "Volts^2", w558, "Volts^3", "Temperature") -> (w562:string)
            }
            frame "Pulsed Wire" {
              w570 = "\t"
              n210 = for {
                tunnel: w575 -> [w582] mode=indexing
                tunnel: [w580] -> w573 mode=indexing
                n211 = Unbundle By Name(w582) -> ("t/f"=w581:bool)
                n212 = Select(t="NaN not included", s=w581, f="") -> (s? t:f=w580:string)
              }
              n213 = Concatenate Strings("Velocity or Tau" ("string"), w570, "1/TOF", w570, "(1/TOF)^2", w570, "(1/TOF)^3", w570, "Temperature") -> (w576:string)
            }
            frame "Generic BackPoly" {
              n214 = global read "Calib_global.vi" "calib units"() -> (w583:string)
              n215 = for {
                tunnel: w585 -> [w593] mode=indexing
                tunnel: [w591] -> w584 mode=indexing
                n216 = Unbundle By Name(w593) -> ("t/f"=w592:bool)
                n217 = Select(t="NaN not included", s=w592, f="") -> (s? t:f=w591:string)
              }
              n218 = Concatenate Strings(w583, "\t", "Voltage") -> (w586:string)
            }
            frame "Fast FID" {
              w595 = "\t"
              n219 = for {
                tunnel: w598 -> [w605] mode=indexing
                tunnel: [w603] -> w597 mode=indexing
                n220 = Unbundle By Name(w605) -> ("t/f"=w604:bool)
                n221 = Select(t="NaN not included", s=w604, f="") -> (s? t:f=w603:string)
              }
              n222 = Concatenate Strings("Concentration (ppm)" ("Substring"), w595, "Voltage", w595, "Stand dev" ("string")) -> (w599:string)
            }
            frame "Thermocouple" {
              n223 = for {
                tunnel: w608 -> [w616] mode=indexing
                tunnel: [w614] -> w607 mode=indexing
                n224 = Unbundle By Name(w616) -> ("t/f"=w615:bool)
                n225 = Select(t="NaN not included", s=w615, f="") -> (s? t:f=w614:string)
              }
              n226 = Concatenate Strings("Temperature", "\t", "Voltage") -> (w609:string)
            }
            frame "Cold wire" {
              n227 = for {
                tunnel: w619 -> [w627] mode=indexing
                tunnel: [w625] -> w618 mode=indexing
                n228 = Unbundle By Name(w627) -> ("t/f"=w626:bool)
                n229 = Select(t="NaN not included", s=w626, f="") -> (s? t:f=w625:string)
              }
              n230 = Concatenate Strings("Temperature", "\t", "Voltage") -> (w620:string)
            }
          }
          n231 = Number To Exponential String(number=w480, precision (6)=i16 10) -> (E-format string=w479:string[][])  [unwired: 2 out]
          n232 = Build Array (concatenate)(w479, w478) -> (w477:string[][])
          n233 = Transpose 2D Array(2D array=w477) -> (transposed array=w476:string[][])
          n234 = call "2D_array_to_string.vi"("2D data array"=w476, "Column titles  (separated by tabs)"=w484, "Array title"="Calib points label") -> ("Output string"=w483:string)
        }
        frame #5 {
          n235 = case shown="\"Cross wire angle\"" w628 {
            tunnel: [w636 w643] -> w629
            tunnel: w630 -> [w635 w643]
            frame "Cross wire angle" {
              w634 = "\r"
              w640 = "Voltage"
              w641 = "\t"
              n236 = global read "Calib_global.vi" "orig vel calib points"() -> (w631:dbl[][])
              n237 = Concatenate Strings("Velocity (m/s)", w641, w640, w641, w640) -> (w638:string)
              n238 = Number To Exponential String(number=w631, precision (6)=10) -> (E-format string=w633:string[][])  [unwired: 2 out]
              n239 = call "2D_array_to_string.vi"("2D data array"=w633, "Column titles  (separated by tabs)"=w638, "Array title"="Original vel calib points") -> ("Output string"=w637:string)
              n240 = Concatenate Strings(w634, w635, w634, w634, w637) -> (w636:string)
            }
            frame "Generic Linear", Default {
            }
          }
        }
        frame #6 {
          n241 = global read "Calib_global.vi" "aux calib file string"() -> (w653:string)
          n242 = call "Add_label_to_string.vi"("String to write"=w653, "File Label"="Auxiliary constants") -> ("Output string"=w656:string)
          n243 = global read "Calib_global.vi" "Instument setup Info"() -> (w645:string)
          n244 = Concatenate Strings(w651, w650, w649, w645, w646, w647) -> (w648:string)
          n245 = case shown="\"Pulsed Wire\"" w652 {
            tunnel: [w658 w667 w672 w678 w690 w695 w700 w711 w721 w732 w737 w742] -> w654
            tunnel: w656 -> [_ _ _ w677 w685 _ _ _ _ _ _ _]
            tunnel: " calib label" -> [w661 w664 w669 _ _ w692 w697 w708 w718 w729 w734 w739]
            tunnel: w648 -> [w660 w663 w668 w674 w683 w691 w696 w703 w717 w726 w733 w738]
            tunnel: "\r" -> [_ _ _ w673 w682 _ _ _ _ _ _ _]
            frame "Propeller anemometer" {
              n246 = Concatenate Strings("Prop", w661) -> (w659:string)
              n247 = call "Add_label_to_string.vi"("String to write"=w660, "File Label"=w659) -> ("Output string"=w658:string)
            }
            frame "Pressure Transducer" {
              n248 = Concatenate Strings("Mano", w664) -> (w665:string)
              n249 = call "Add_label_to_string.vi"("String to write"=w663, "File Label"=w665) -> ("Output string"=w667:string)
            }
            frame "Hot wire" {
              n250 = Concatenate Strings("HW", w669) -> (w671:string)
              n251 = call "Add_label_to_string.vi"("String to write"=w668, "File Label"=w671) -> ("Output string"=w672:string)
            }
            frame "Cross wire velocity" {
              n252 = global read "Calib_global.vi" "Angle/vel calib file string"() -> (w675:string)
              n253 = call "Add_label_to_string.vi"("String to write"=w674, "File Label"="Cross wire velocity calib label") -> ("Output string"=w679:string)
              n254 = call "Add_label_to_string.vi"("String to write"=w675, "File Label"="Cross wire angle calib label") -> ("Output string"=w676:string)
              n255 = Concatenate Strings(w679, w673, w677, w673, w673, w676) -> (w678:string)
            }
            frame "Cross wire angle" {
              n256 = global read "Calib_global.vi" "Angle/vel calib file string"() -> (w684:string)
              n257 = call "Add_label_to_string.vi"("String to write"=w684, "File Label"="Cross wire velocity calib label") -> ("Output string"=w687:string)
              n258 = call "Add_label_to_string.vi"("String to write"=w683, "File Label"="Cross wire angle calib label") -> ("Output string"=w686:string)
              n259 = Concatenate Strings(w687, w682, w685, w682, w682, w686) -> (w690:string)
            }
            frame "Generic Linear" {
              n260 = Concatenate Strings("Generic Inst", w692) -> (w693:string)
              n261 = call "Add_label_to_string.vi"("String to write"=w691, "File Label"=w693) -> ("Output string"=w695:string)
            }
            frame "Generic Polynomial" {
              n262 = Concatenate Strings("Generic Polynomial", w697) -> (w698:string)
              n263 = call "Add_label_to_string.vi"("String to write"=w696, "File Label"=w698) -> ("Output string"=w700:string)
            }
            frame "Pulsed Wire" {
              n264 = global read "PWAtasksGLOBAL.vi" "PWA Lookup Table"() -> (w707:dbl[])
              n265 = for {
                tunnel: w707 -> [w716] mode=indexing
                shift-right: [w712] -> w705
                shift-left: "" -> [w713]
                n266 = Number To Exponential String(number=w716) -> (E-format string=w714:string)  [unwired: 3 out]
                n267 = Concatenate Strings(w713, w714, "\r") -> (w712:string)
              }
              n268 = Concatenate Strings("Pulsed wire", w708) -> (w709:string)
              n269 = call "Add_label_to_string.vi"("String to write"=w705, "File Label"="Pulsed_wire_lookup_table") -> ("Output string"=w702:string)
              n270 = Concatenate Strings(w703, w702) -> (w701:string)
              n271 = call "Add_label_to_string.vi"("String to write"=w701, "File Label"=w709) -> ("Output string"=w711:string)
            }
            frame "Generic BackPoly" {
              n272 = Concatenate Strings("Generic BackPoly", w718) -> (w719:string)
              n273 = call "Add_label_to_string.vi"("String to write"=w717, "File Label"=w719) -> ("Output string"=w721:string)
            }
            frame "Fast FID" {
              n274 = Concatenate Strings("Fast FID", w729) -> (w730:string)
              n275 = call "Replace_data_in_setup_string.vi"("New data string"="0.00", "Input string"=w726, "Variable name"="Fast FID Bkgnd") -> ("Appended string"=w723:string)
              n276 = call "Replace_data_in_setup_string.vi"("New data string"="0.00", "Input string"=w723, "Variable name"="Fast FID Bkgnd Variance") -> ("Appended string"=w722:string)
              n277 = call "Add_label_to_string.vi"("String to write"=w722, "File Label"=w730) -> ("Output string"=w732:string)
            }
            frame "Thermocouple" {
              n278 = Concatenate Strings("Thermocouple", w734) -> (w735:string)
              n279 = call "Add_label_to_string.vi"("String to write"=w733, "File Label"=w735) -> ("Output string"=w737:string)
            }
            frame "Cold wire" {
              n280 = Concatenate Strings("Cold wire", w739) -> (w740:string)
              n281 = call "Add_label_to_string.vi"("String to write"=w738, "File Label"=w740) -> ("Output string"=w742:string)
            }
          }
          n282 = global write "Calib_global.vi" "Header string"(w654) -> ()
        }
      }
    }
    frame #5 {
      n283 = local read "Point selector 4"() -> (→"Point selector 4 out":T1)
      n284 = local read "Point selector 3"() -> (→"Point selector 3 out":cluster{"Y":dbl, "X":dbl, "t/f":bool}[])
    }
  }
